vi "Actor Core.vi"(8 "error in":errorcluster, 11 "Calculator Actor in":refnum<class "Calculator Actor.lvclass">) -> (0 "error out":errorcluster, 3 "Actor out":refnum<class "Actor.lvclass">)   [LabVIEW 2014, in "Calculator Actor.lvclass"]
doc: "(<B>Filename</B>: Actor Framework.lvlib:Actor.lvclass:Actor Core.vi)\n\nReceives messages to the actor, reacts to them, and initiates any error handling that may shut the actor down.\n\nDescendant classes may override this VI to append parallel tasks for the actor to complete while it handles messages. Overrides use the Call Parent Method node."
uses:
  Calculator Actor.lvclass
  <vilib>/ActorFramework/Actor/Actor.lvclass
  Addition Actor/Addition Actor Class/Addition Actor.lvclass
  Multiplication Actor/Multiplication Actor Class/Multiplication Actor.lvclass
  Calculator Actor.lvclass/Calculator Actor.ctl
  <vilib>/ActorFramework/Actor/Actor.lvclass/Actor.ctl
  <vilib>/ActorFramework/Message Enqueuer/Message Enqueuer.lvclass/Message Enqueuer.ctl
  <vilib>/ActorFramework/Message Enqueuer/Init from Existing Queue.vi
  <vilib>/ActorFramework/Message Enqueuer/Enqueue.vi
  <vilib>/ActorFramework/Message Priority Queue/Priority Enqueue.vi
  <vilib>/ActorFramework/Message Enqueuer/Message Enqueuer.lvclass
  <vilib>/ActorFramework/Stop Msg/Stop Msg.lvclass
  Multiplication Actor/Multiplication Actor Messages/Multiplication Request Msg/Multiplication Request Msg.lvclass
  Addition Actor/Addition Actor Messages/Addition Request Msg/Addition Request Msg.lvclass
panel:
  in  "Calculate":bool
  out "Result - Multiplication":dbl
  out "Result - Addition":dbl
  in  "Number 2":dbl
  in  "Number 1":dbl
  in  "stop":bool
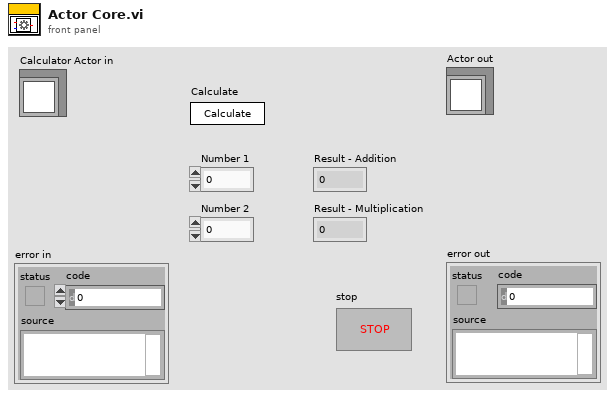
[diagram p1: front panel]
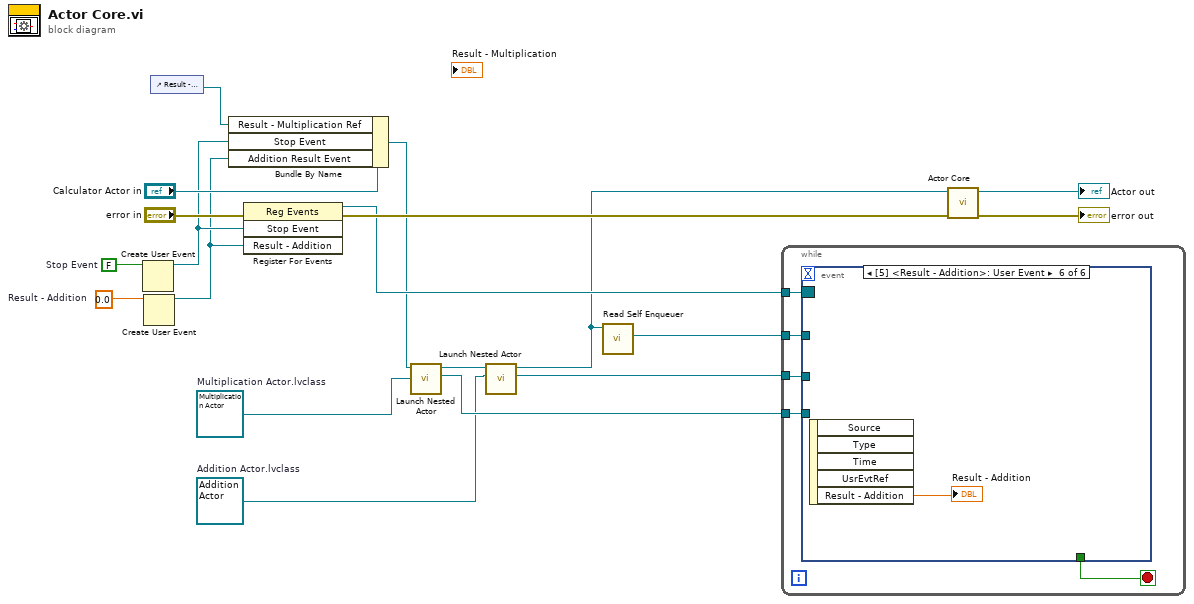
[diagram p0: block diagram]
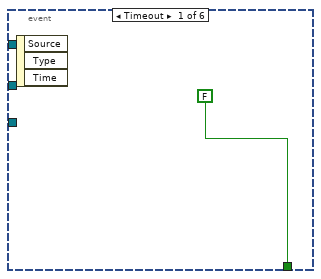
[diagram p2: hidden frame]
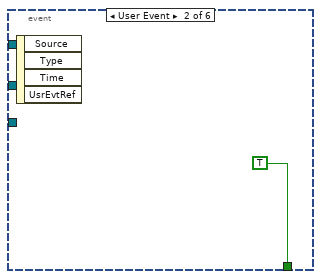
[diagram p3: hidden frame]
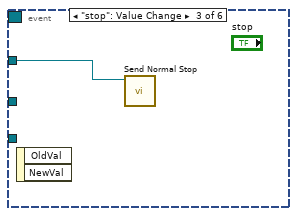
[diagram p4: hidden frame]
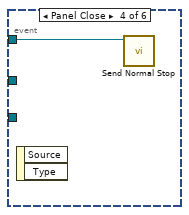
[diagram p5: hidden frame]
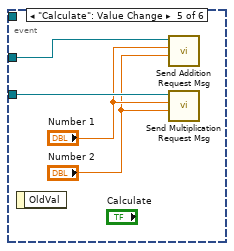
[diagram p6: hidden frame]
diagram:
  w3 = 0.0  # Result - Addition
  w5 = refnum<class "Multiplication Actor.lvclass"> refnum  # Multiplication Actor.lvclass
  w4 = refnum<class "Addition Actor.lvclass"> refnum  # Addition Actor.lvclass
  w14 = FALSE  # Stop Event
  n1 = Create User Event(user event datatype=w14) -> (user event=w12:refnum<user-event>)  [unwired: 1 in, 1 out]
  n2 = Create User Event(user event datatype=w3) -> (user event=w2:refnum<user-event>)  [unwired: 1 in, 1 out]
  n3 = control-ref of="Result - Multiplication"() -> (w1:refnum<vi>)
  n4 = Bundle By Name(cluster="Calculator Actor in", "Result - Multiplication Ref"=w1, "Stop Event"=w12, "Addition Result Event"=w2) -> (w9:refnum<class "Calculator Actor.lvclass">)
  n5 = register-events(error in="error in", w12, w2) -> (reference out=w15:refnum<event-registration>, error out=w16:errorcluster)  [unwired: 1 in]
  n6 = call <vilib>:"Launch Nested Actor.vi"("Nested Actor"=w5, "Caller Actor in"=w9) -> ("Nested Actor's Enqueuer"=w6:refnum<class "Message Enqueuer.lvclass">, "Caller Actor out"=w10:refnum<class "Calculator Actor.lvclass">)  [unwired: 7 in, 1 out]
  n7 = call <vilib>:"Launch Nested Actor.vi"("Nested Actor"=w4, "Caller Actor in"=w10) -> ("Nested Actor's Enqueuer"=w7:refnum<class "Message Enqueuer.lvclass">, "Caller Actor out"=w8:refnum<class "Calculator Actor.lvclass">)  [unwired: 7 in, 1 out]
  n8 = call <vilib>:"Read Self Enqueuer.vi"("Actor"=w8) -> ("Self Enqueuer"=w11:refnum<class "Message Enqueuer.lvclass">)  [unwired: 10 in]
  n9 = while {
    tunnel: w15 -> [w24]
    tunnel: w11 -> [w22]
    tunnel: w7 -> [w21]
    tunnel: w6 -> [w20]
    stop <- w23 stop-if-true
    n10 = event shown="[5] <Result - Addition>: User Event" {
      selector: w24 -> [_ _ _ _ _ _]
      dyn-events: _ -> [_ _ _ _ _ _]
      timeout: _ -> [_ _ _ _ _ _]
      tunnel: [FALSE TRUE _ _ _ _] -> w23
      tunnel: w22 -> [_ _ w27 w28 _ _]
      tunnel: w21 -> [_ _ _ _ w31 _]
      tunnel: w20 -> [_ _ _ _ w32 _]
      event Timeout {
        n11 = event-data() -> ()  [unwired: 1 in, 3 out]
      }
      event User Event {
        n12 = event-data() -> ()  [unwired: 1 in, 4 out]
      }
      event "stop": Value Change {
        n13 = event-data() -> ()  [unwired: 1 in, 2 out]
        n14 = call <vilib>:"Send Normal Stop.vi"("Message Enqueuer"=w27) -> ()  [unwired: 10 in, 1 out]
      }
      event Panel Close {
        n15 = event-data() -> ()  [unwired: 1 in, 2 out]
        n16 = call <vilib>:"Send Normal Stop.vi"("Message Enqueuer"=w28) -> ()  [unwired: 10 in, 1 out]
      }
      event "Calculate": Value Change {
        n17 = event-data() -> ()  [unwired: 1 in, 1 out]
        n18 = call "Send Addition Request Msg.vi"("Number 2"="Number 2", "Number 1"="Number 1", "Message Enqueuer in"=w31) -> ()  [unwired: 7 in, 2 out]
        n19 = call "Send Multiplication Request Msg.vi"("Number 2"="Number 2", "Number 1"="Number 1", "Message Enqueuer in"=w32) -> ()  [unwired: 7 in, 2 out]
      }
      event User Event {
        n20 = event-data() -> ("Result - Addition"=→"Result - Addition":dbl)  [unwired: 1 in, 4 out]
      }
    }
  }
  n21 = call-parent "Actor Core.vi"("error in"=w16, "Actor in"=w8) -> ("error out"=→"error out":errorcluster, "Actor out"=→"Actor out":refnum<class "Actor.lvclass">)  [unwired: 8 in]
